vi "Teleop Drive V.5.0.vi"   [LabVIEW 2016]
uses:
  <vilib>/Rock Robotics/WPI/ThirdParty/CanMotor/TalonSRX/WPI_CANTalonSRX_BrakeOverride.ctl
  Robot Global Data V.5.0.vi
  <vilib>/Rock Robotics/WPI/Utilities/WPI_GetSetVariantRefNum.vi
  <vilib>/Rock Robotics/WPI/RobotDrive/WPI_RobotDriveArcadeDrive_Standard(NoSaturation).vi
  <vilib>/Rock Robotics/Network Tables/NT Write Numeric Array.vi
types:
  T1 = typedef "WPI_CANTalonSRX_BrakeOverride.ctl" = enum8{"No Override", "Override to Coast", "Override to Brake"}
  T2 = typedef "WPI_RobotDriveDevRef.ctl" = cluster{"DevStatus":errorcluster, "Motors[]":T3[], "Square Inputs":bool, "Max Output":dbl}
  T3 = typedef "WPI_MotorControlDeviceRef.ctl" = cluster{"DeviceStatus":errorcluster, "Type":T4, "PWM":cluster{"PWM Channel":T5, "DeadBand":T6}, "CAN":cluster{"Device Number":u8, "SetOutput VI Ref":variant, "GetOutput VI Ref":variant, "Enable VI Ref":variant, "Disable VI Ref":variant, "Data":variant}, "Invert":bool}
  T4 = typedef "WPI_MotorControlType.ctl" = enum16{"PWM", "CAN"}
  T5 = typedef "FPGA_DIOPWMChannel.ctl" = enum8{"PWM 0", "PWM 1", "PWM 2", "PWM 3", "PWM 4", "PWM 5", "PWM 6", "PWM 7", "PWM 8", "PWM 9", "PWM MXP 0", "PWM MXP 1", "PWM MXP 2", "PWM MXP 3", "PWM MXP 4", "PWM MXP 5", "PWM MXP 6", "PWM MXP 7", "PWM MXP 8", "PWM MXP 9", "Invalid"}
  T6 = typedef "WPI_PWMDeadband.ctl" = cluster{"Name":string, "maxPositivePwm":i32, "minPositivePwm":i32, "centerPwm":i32, "maxNegativePwm":i32, "minNegativePwm":i32, "angularRange":u16}
  T7 = typedef "WPI_CANTalonSRX_GlobalStatus.ctl" = cluster{"Applied Throttle":dbl, "Module Enabled":bool, "CAN Error":errorcluster, "Closed Loop Error":dbl, "Forward Limit Switch Closed":bool, "Reverse Limit Switch Closed":bool, "Sensor Position":dbl, "Sensor Velocity":dbl, "Current":dbl, "Sticky Fault - Over Temp":bool, "Sticky Fault - Under Voltage":bool, "Sticky Fault - Forward Limit":bool, "Sticky Fault - Reverse Limit":bool, "Sticky Fault - Forward Soft Limit":bool, "Sticky Fault - Reverse Soft Limit":bool, "Brake is Enabled":bool, "Encoder Position":dbl, "Encoder Velocity":dbl, "Encoder Index Count":dbl, "Encoder A Pin State":bool, "Encoder B Pin State":bool, "Encoder Index Pin State":bool, "Analog In":dbl, "Analog In Velocity":dbl, "Temperature (C)":dbl, "Battery Voltage":dbl, "Control 5 Is Supported":bool, "Current Profile Slot Select":dbl, "Pos Div 8":bool, "Vel Div 4":bool, "Pulse Width Position":i32, "Pulse Width Velocity":i32, "Pulse Width Rise To Rise (us)":i32, "Pulse Width Rise To Fall (us)":i32, "Mot Prof Active Is Under Run":bool, "Mot Prof Active Has Under Run":bool, "Mot Prof Active Is Last":bool, "Mot Prof Active Velocity Only":bool, "Mot Prof Active Is Valid":bool, "Mot Prof Buffer Is Full":bool, "Mot Prof Active Profile Slot Select":i32, "Mot Prof NextID":i32, "Mot Prof Count":i32, "Mot Prof Active Velocity":dbl, "Mot Prof Active Position":dbl, "Mot Prof Output Enable":i32}
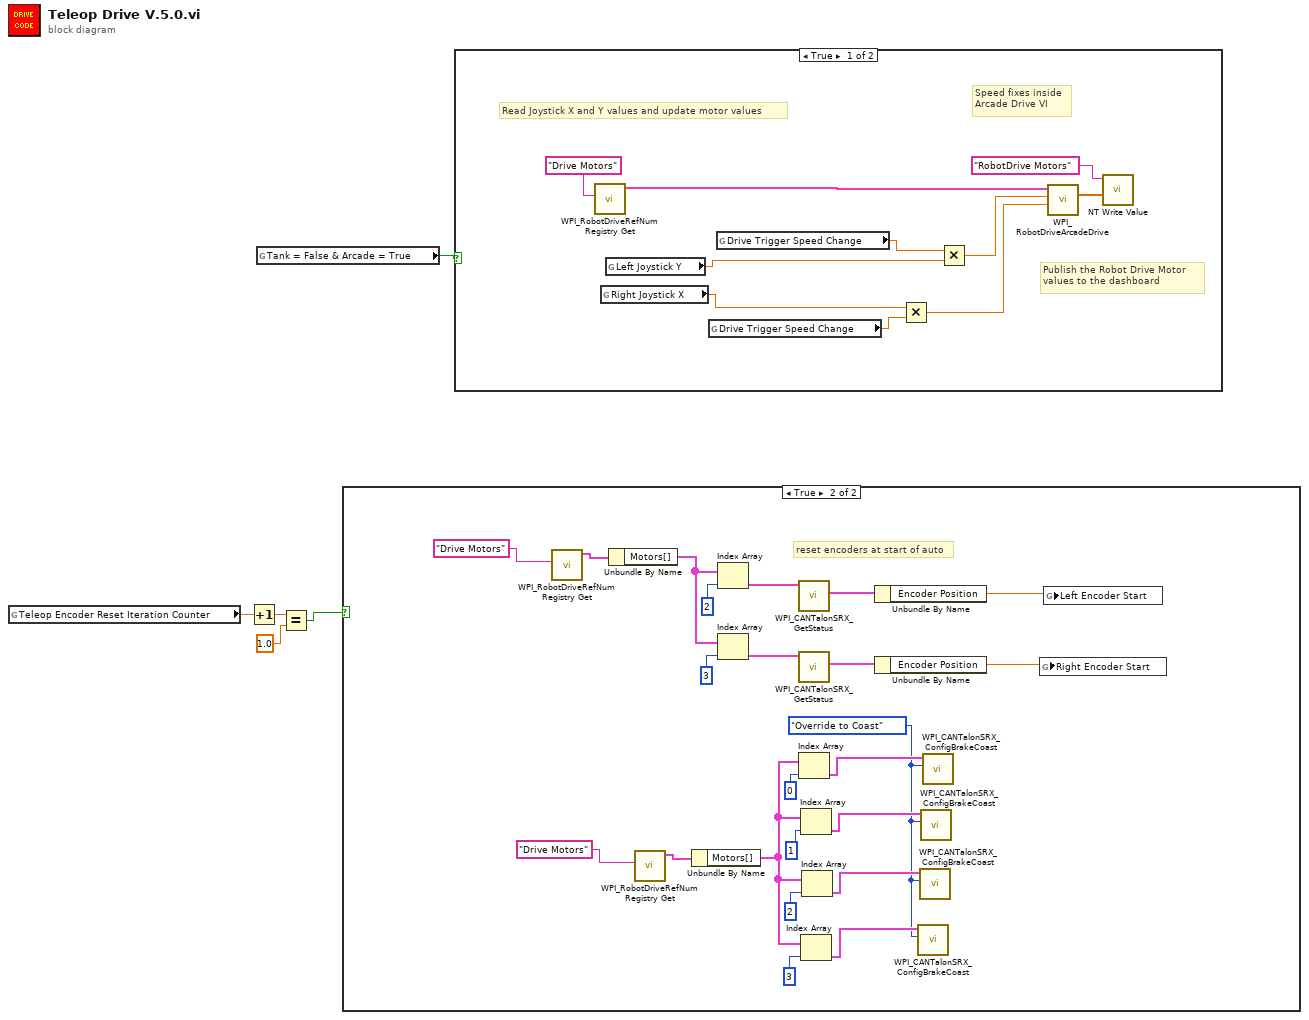
[diagram p0: block diagram]
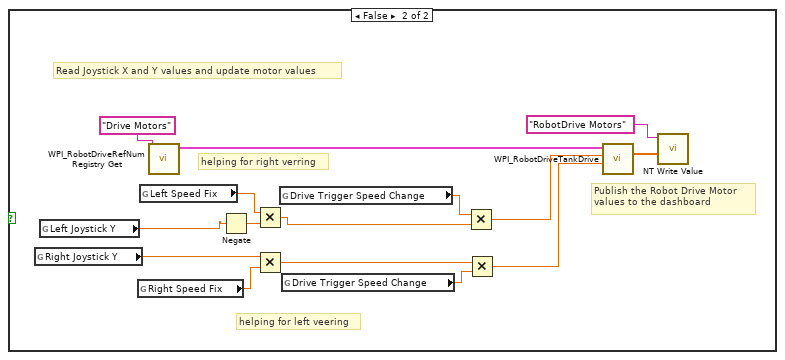
[diagram p3: hidden frame]
diagram:
  n1 = global read "Robot Global Data V.5.0.vi" "Teleop Encoder Reset Iteration Counter"() -> (w4:dbl)
  n2 = Increment(x=w4) -> (x+1=w3:dbl)
  n3 = global read "Robot Global Data V.5.0.vi" "Tank = False & Arcade = True"() -> (w5:bool)
  n4 = Equal?(x=w3, y=1.0) -> (x = y?=w1:bool)
  n5 = case shown="True" w1 {
    frame False {
    }
    frame True {
      w6 = WPI_CANTalonSRX_BrakeOverride."Override to Coast" ("Brake / Coast Mode")
      # "reset encoders at start of auto"
      n6 = call <vilib>:"WPI_RobotDriveRefNum Registry Get.vi"("refnum name"="Drive Motors") -> ("RobotDriveDevRef"=w27:T2)  [unwired: 9 in, 1 out]
      n7 = Unbundle By Name(w27) -> ("Motors[]"=w18:T3[])
      n8 = call <vilib>:"WPI_RobotDriveRefNum Registry Get.vi"("refnum name"="Drive Motors") -> ("RobotDriveDevRef"=w16:T2)  [unwired: 9 in, 1 out]
      n9 = Unbundle By Name(w16) -> ("Motors[]"=w11:T3[])
      n10 = Index Array(array=w18, index=2) -> (element=w25:T3)
      n11 = Index Array(array=w18, index=3) -> (element=w21:T3)
      n12 = call <vilib>:"WPI_CANTalonSRX_GetStatus.vi"("CAN Talon SRX Ref"=w25) -> ("Talon SRX Status"=w24:T7)  [unwired: 8 in, 2 out]
      n13 = call <vilib>:"WPI_CANTalonSRX_GetStatus.vi"("CAN Talon SRX Ref"=w21) -> ("Talon SRX Status"=w20:T7)  [unwired: 8 in, 2 out]
      n14 = Index Array(array=w11, index=0) -> (element=w10:T3)
      n15 = Index Array(array=w11, index=1) -> (element=w9:T3)
      n16 = Index Array(array=w11, index=3) -> (element=w7:T3)
      n17 = Index Array(array=w11, index=2) -> (element=w8:T3)
      n18 = Unbundle By Name(w24) -> ("Encoder Position"=w23:dbl)
      n19 = Unbundle By Name(w20) -> ("Encoder Position"=w19:dbl)
      n20 = call <vilib>:"WPI_CANTalonSRX_ConfigBrakeCoast.vi"("Brake / Coast Mode"=w6, "CAN Talon SRX Ref"=w7) -> ()  [unwired: 8 in, 2 out]
      n21 = call <vilib>:"WPI_CANTalonSRX_ConfigBrakeCoast.vi"("Brake / Coast Mode"=w6, "CAN Talon SRX Ref"=w8) -> ()  [unwired: 8 in, 2 out]
      n22 = call <vilib>:"WPI_CANTalonSRX_ConfigBrakeCoast.vi"("Brake / Coast Mode"=w6, "CAN Talon SRX Ref"=w9) -> ()  [unwired: 8 in, 2 out]
      n23 = call <vilib>:"WPI_CANTalonSRX_ConfigBrakeCoast.vi"("Brake / Coast Mode"=w6, "CAN Talon SRX Ref"=w10) -> ()  [unwired: 8 in, 2 out]
      n24 = global write "Robot Global Data V.5.0.vi" "Right Encoder Start"(w19) -> ()
      n25 = global write "Robot Global Data V.5.0.vi" "Left Encoder Start"(w23) -> ()
    }
  }
  n26 = case shown="True" w5 {
    frame True {
      # "Speed fixes inside \nArcade Drive VI"
      # "Publish the Robot Drive Motor\nvalues to the dashboard"
      # "Read Joystick X and Y values and update motor values"
      n27 = call <vilib>:"WPI_RobotDriveRefNum Registry Get.vi"("refnum name"="Drive Motors") -> ("RobotDriveDevRef"=w37:T2)  [unwired: 1 in, 9 out]
      n28 = global read "Robot Global Data V.5.0.vi" "Right Joystick X"() -> (w30:dbl)
      n29 = global read "Robot Global Data V.5.0.vi" "Left Joystick Y"() -> (w33:dbl)
      n30 = global read "Robot Global Data V.5.0.vi" "Drive Trigger Speed Change"() -> (w31:dbl)
      n31 = global read "Robot Global Data V.5.0.vi" "Drive Trigger Speed Change"() -> (w34:dbl)
      n32 = Multiply(x=w30, y=w31) -> (x*y=w29:dbl)
      n33 = Multiply(x=w34, y=w33) -> (x*y=w32:dbl)
      n34 = call-poly <vilib>:"WPI_RobotDriveArcadeDrive.vi"("Y axis value"=w29, "X axis value"=w32, "RobotDriveDevRef"=w37) -> ("Motor Values"=w36:dbl[])  [unwired: 6 in, 2 out]
      n35 = call-poly <vilib>:"NT Write Value.vi"("Numeric Array"=w36, "Name"="RobotDrive Motors") -> ()  [unwired: 9 in, 1 out]
    }
    frame False {
      # "helping for left veering"
      # "helping for right verring"
      # "Publish the Robot Drive Motor\nvalues to the dashboard"
      # "Read Joystick X and Y values and update motor values"
      n36 = global read "Robot Global Data V.5.0.vi" "Right Joystick Y"() -> (w45:dbl)
      n37 = global read "Robot Global Data V.5.0.vi" "Left Joystick Y"() -> (w49:dbl)
      n38 = global read "Robot Global Data V.5.0.vi" "Right Speed Fix"() -> (w46:dbl)
      n39 = global read "Robot Global Data V.5.0.vi" "Left Speed Fix"() -> (w47:dbl)
      n40 = call <vilib>:"WPI_RobotDriveRefNum Registry Get.vi"("refnum name"="Drive Motors") -> ("RobotDriveDevRef"=w52:T2)  [unwired: 1 in, 9 out]
      n41 = Negate(x=w49) -> (-x=w48:dbl)
      n42 = Multiply(x=w47, y=w48) -> (x*y=w43:dbl)
      n43 = Multiply(x=w45, y=w46) -> (x*y=w39:dbl)
      n44 = global read "Robot Global Data V.5.0.vi" "Drive Trigger Speed Change"() -> (w44:dbl)
      n45 = global read "Robot Global Data V.5.0.vi" "Drive Trigger Speed Change"() -> (w40:dbl)
      n46 = Multiply(x=w44, y=w43) -> (x*y=w42:dbl)
      n47 = Multiply(x=w39, y=w40) -> (x*y=w41:dbl)
      n48 = call <vilib>:"WPI_RobotDriveTankDrive.vi"("Right axis value"=w41, "Left axis value"=w42, "RobotDriveDevRef"=w52) -> ("Motor Values"=w51:dbl[])  [unwired: 6 in, 2 out]
      n49 = call-poly <vilib>:"NT Write Value.vi"("Numeric Array"=w51, "Name"="RobotDrive Motors") -> ()  [unwired: 9 in, 1 out]
    }
  }
